vi "Start Run.vi"(6 "clone#":i32, 8 "done ref":refnum<vi>, 11 "target in":refnum<class "Base Target.lvclass">) -> (3 "target out":refnum<class "Base Target.lvclass">)   [LabVIEW 2020, in "NI_TargetHelper.lvlib" / "Base Target.lvclass"]
uses:
  <vilib>/TargetSupport/NI_TargetHelper/Base Target/Base Target.lvclass
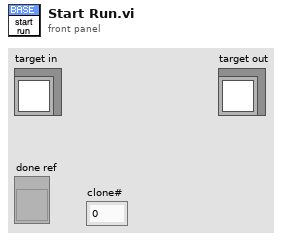
[diagram p1: front panel]
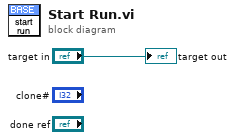
[diagram p0: block diagram]
diagram:
  "target out" <- "target in"
